vi "ECAT Wipeback FoE.vi"(8 "error in":errorcluster, 11 "FoE Command":string) -> (0 "error out":errorcluster, 3 "Output byte array":u8[](array[numeric]))   [LabVIEW 2020, in "SEECD System Explorer.lvlib"]
uses:
  SEECD System Explorer.lvlib
  <vilib>/Utility/sysdir.llb/Get System Directory.vi
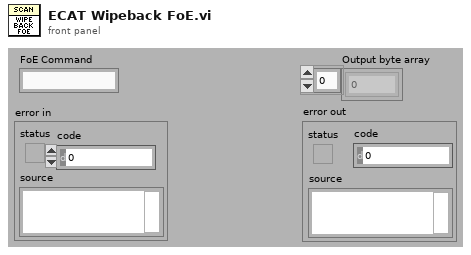
[diagram p1: front panel]
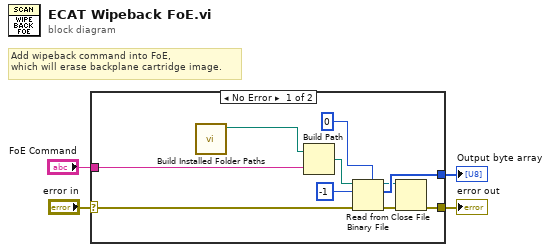
[diagram p0: block diagram]
diagram:
  # "Add wipeback command into FoE,\nwhich will erase backplane cartridge image."
  n1 = case shown="No Error" "error in" {
    selector: "error in" -> [w11 w15]
    tunnel: [w12 _] -> w4
    tunnel: [w8 w15] -> w3
    tunnel: "FoE Command" -> [w7 _]
    frame No Error {
      n2 = call "Build Installed Folder Paths.vi"() -> ("Data Folder Path"=w6:path)  [unwired: 10 in, 1 out]
      n3 = Build Path(base path=w6, name or relative path=w7) -> (appended path=w5:path)
      n4 = Read from Binary File(5:u8 0, 8:w11, 10:-1 ("count (1)"), 11:w5) -> (0:w9:errorcluster, 2:w12:u8[], 3:w10:refnum<file>)  [unwired: 2 in, 1 out]
      n5 = Close File(refnum=w10, error in=w9) -> (error out=w8:errorcluster)  [unwired: 1 out]
    }
    frame Error {
    }
  }
  "error out" <- w3
  "Output byte array" <- w4
